vi "Get Unique Test ID.vi"(1 "board in":refnum<class "Board Design.lvclass">) -> (0 "id #":u32)   [LabVIEW 2023, in "Board Design.lvclass"]
doc: "Get an identification number."
uses:
  Board Design.lvclass
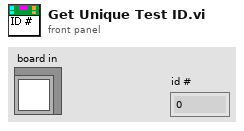
[diagram p1: front panel]
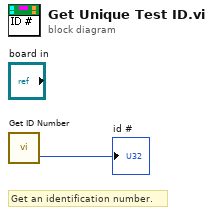
[diagram p0: block diagram]
diagram:
  # "Get an identification number."
  n1 = call "Get ID Number.vi"() -> ("id number"=→"id #":u32)  [unwired: 2 in]
